vi "Verarbeitung_Oben.vi"(8 "Fehler in":errorcluster, 10 "Größe Kontaktsuchfeld":sgl=50.0, 11 "Cluster in":T1={"Initialisierung"={"Online?"=FALSE, "Grundpfad"=path "", "Kamera Oben"="", "IP-Adresse Flüssiglinse"="", "Flüssiglinse"=refnum, "Kamera Unten"="", "IP-Adresse SPS"="", "SPS-Verbindung"={"TCP Connection Ref"=refnum, "IP address"="", "timeout ms"=5000, "Connected?"=FALSE, "PLC Type"=enum."S7 1200", "Rack S7 400"=0, "Slot S7 400"=0, "PDU Size"=0, "connection semaphore"=refnum}, "IP-Adresse Lichtgitter"="", "Lichtgitter"=refnum, "Skalierungsfaktor"=0.0, "Bilder Oben"=[], "Bild Unten"=refnum, "Bild Ausschnitt Unten"=refnum}, "Einstellungen"={"Gesamtablauf gestartet"=FALSE, "i. O. Bilder speichern"=FALSE, "Bildspeicherung Offline"=FALSE, "Ausgewähltes Offline-Datum"="", "Ausgewähltes Offline-Teil"="", "Speicherpfad Bilder"=path ""}, "Artikeldaten"={"Artikelnummer"="", "Fertigungsauftrag"="", "Muster ISO"=refnum, "Belichtungszeit Referenzmarken"=0.0, "Fokus Referenzmarken"=0.0, "Belichtungszeit ISO"=0.0, "Fokus ISO"=0.0, "Belichtungszeit Unten"=0.0, "Kontaktanzahl"=0, "Aktueller Kontakt"=0, "Kontaktposition"={"x"=0.0, "y"=0.0}, "Winkel ISO"=0.0, "ISO-Muster nicht vorhanden"=FALSE}, "Werte Kamera Oben"={"Koordinatensystem"={"Punkt x-Achse"={"X"=0.0, "Y"=0.0}, "Ursprung"={"X"=0.0, "Y"=0.0}, "Punkt y-Achse"={"X"=0.0, "Y"=0.0}}, "Position Kontakt"={"x"=0.0, "y"=0.0}, "Winkel Kontakt"=0.0}, "Werte Kamera Unten"={"Prüfung Unten n. i. O."=FALSE}, "Werte Lichtgitter"={"Messwerte Referenzmarken"=[], "Mittelpunkt Referenzmarken"={"x"=0.0, "y"=0.0}, "Messwerte Kontakt"=[], "Offset"={"x"=0.0, "y"=0.0}}, "Rückmeldungen"={"Koordinaten ermittelt"=FALSE, "Vermessung Lichtgitter fertig"=FALSE, "Nachkontrolle Kamera Unten fertig"=FALSE}, "Fehler"={"Referenzen nicht gefunden"=FALSE, "Kontakt nicht gefunden"=FALSE, "Referenzen nicht in Lichtgitter"=FALSE, "Kontakt zu groß"=FALSE, "Kontakt zu klein"=FALSE}, "Statistik"={"Statistiken"=[]}, "Timer"={"Timer Start Position"=0, "Timer Start Lichtgitter"=0, "Timer Start Kamera Unten"=0}}) -> (0 "Fehler out":errorcluster, 2 "Durchmesser Loch":dbl, 3 "Cluster out":T1={"Initialisierung"={"Online?"=FALSE, "Grundpfad"=path "", "Kamera Oben"="", "IP-Adresse Flüssiglinse"="", "Flüssiglinse"=refnum, "Kamera Unten"="", "IP-Adresse SPS"="", "SPS-Verbindung"={"TCP Connection Ref"=refnum, "IP address"="", "timeout ms"=5000, "Connected?"=FALSE, "PLC Type"=enum."S7 1200", "Rack S7 400"=0, "Slot S7 400"=0, "PDU Size"=0, "connection semaphore"=refnum}, "IP-Adresse Lichtgitter"="", "Lichtgitter"=refnum, "Skalierungsfaktor"=0.0, "Bilder Oben"=[], "Bild Unten"=refnum, "Bild Ausschnitt Unten"=refnum}, "Einstellungen"={"Gesamtablauf gestartet"=FALSE, "i. O. Bilder speichern"=FALSE, "Bildspeicherung Offline"=FALSE, "Ausgewähltes Offline-Datum"="", "Ausgewähltes Offline-Teil"="", "Speicherpfad Bilder"=path ""}, "Artikeldaten"={"Artikelnummer"="", "Fertigungsauftrag"="", "Muster ISO"=refnum, "Belichtungszeit Referenzmarken"=0.0, "Fokus Referenzmarken"=0.0, "Belichtungszeit ISO"=0.0, "Fokus ISO"=0.0, "Belichtungszeit Unten"=0.0, "Kontaktanzahl"=0, "Aktueller Kontakt"=0, "Kontaktposition"={"x"=0.0, "y"=0.0}, "Winkel ISO"=0.0, "ISO-Muster nicht vorhanden"=FALSE}, "Werte Kamera Oben"={"Koordinatensystem"={"Punkt x-Achse"={"X"=0.0, "Y"=0.0}, "Ursprung"={"X"=0.0, "Y"=0.0}, "Punkt y-Achse"={"X"=0.0, "Y"=0.0}}, "Position Kontakt"={"x"=0.0, "y"=0.0}, "Winkel Kontakt"=0.0}, "Werte Kamera Unten"={"Prüfung Unten n. i. O."=FALSE}, "Werte Lichtgitter"={"Messwerte Referenzmarken"=[], "Mittelpunkt Referenzmarken"={"x"=0.0, "y"=0.0}, "Messwerte Kontakt"=[], "Offset"={"x"=0.0, "y"=0.0}}, "Rückmeldungen"={"Koordinaten ermittelt"=FALSE, "Vermessung Lichtgitter fertig"=FALSE, "Nachkontrolle Kamera Unten fertig"=FALSE}, "Fehler"={"Referenzen nicht gefunden"=FALSE, "Kontakt nicht gefunden"=FALSE, "Referenzen nicht in Lichtgitter"=FALSE, "Kontakt zu groß"=FALSE, "Kontakt zu klein"=FALSE}, "Statistik"={"Statistiken"=[]}, "Timer"={"Timer Start Position"=0, "Timer Start Lichtgitter"=0, "Timer Start Kamera Unten"=0}})   [LabVIEW 2024]
doc: "Ermittelt die Position des nächsten Kontakts im Koordinatensystem der Referenzbohrungen."
uses:
  Cluster.ctl
  Kontaktmontagemodul.exe/1abvi3w/vi.lib/userDefined/High Color/IMAQdx.ctl
  Kontaktmontagemodul.exe/1abvi3w/vi.lib/DATA AHEAD/SP7/typedefs/S7 Connection.ctl
  Kontaktmontagemodul.exe/1abvi3w/vi.lib/DATA AHEAD/SP7/typedefs/PLC Type.ctl
  Kontaktmontagemodul.exe/1abvi3w/vi.lib/vision/Image Controls.llb/IMAQ Image.ctl
  Koordinatensystem.ctl
  Statistik.ctl
  Kontaktmontagemodul.exe/1abvi3w/vi.lib/DATA AHEAD/SP7/SP7.lvlib
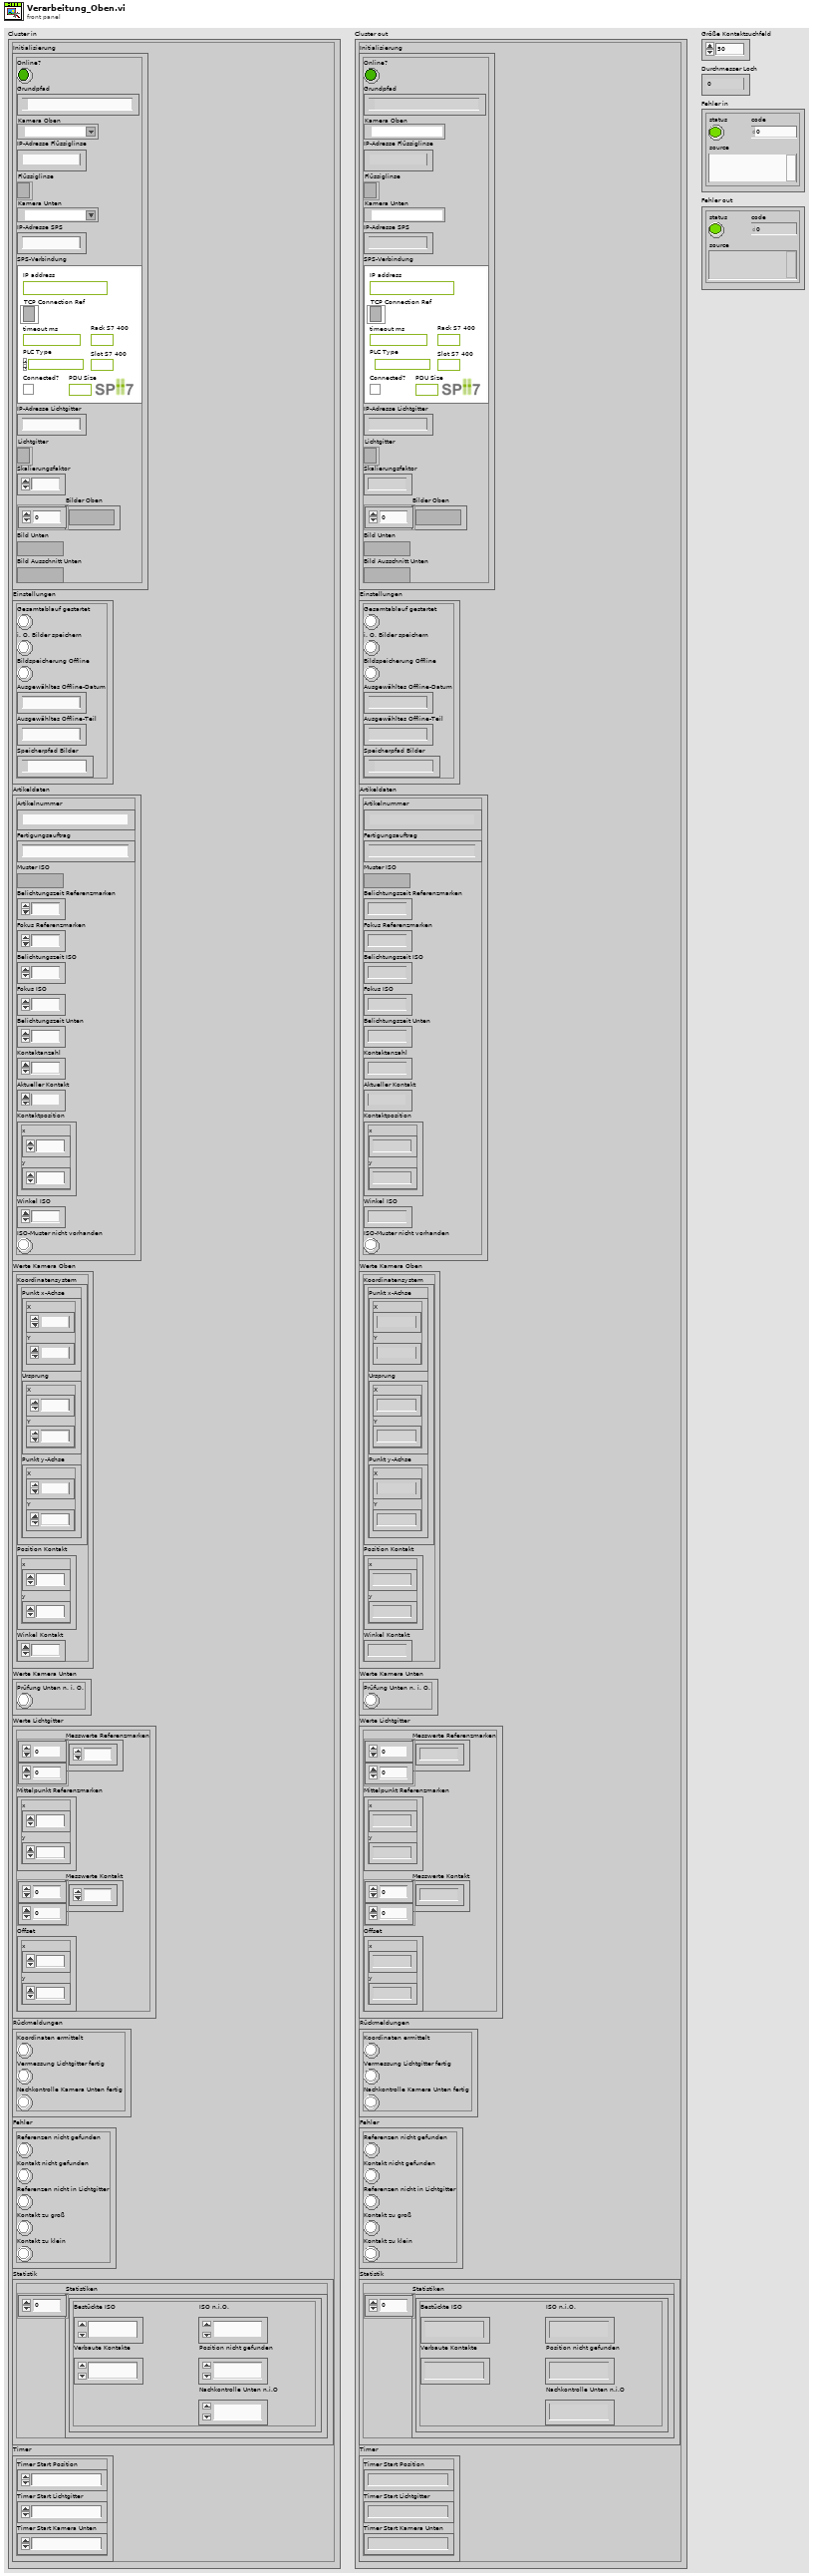
[diagram p1: front panel]
types:
  T1 = typedef "Cluster.ctl" = cluster{"Initialisierung":cluster{"Online?":bool, "Grundpfad":path, "Kamera Oben":T2, "IP-Adresse Flüssiglinse":string, "Flüssiglinse":refnum<k5>, "Kamera Unten":T2, "IP-Adresse SPS":string, "SPS-Verbindung":T3, "IP-Adresse Lichtgitter":string, "Lichtgitter":refnum<k5>, "Skalierungsfaktor":dbl, "Bilder Oben":T6[], "Bild Unten":T6, "Bild Ausschnitt Unten":T6}, "Einstellungen":cluster{"Gesamtablauf gestartet":bool, "i. O. Bilder speichern":bool, "Bildspeicherung Offline":bool, "Ausgewähltes Offline-Datum":string, "Ausgewähltes Offline-Teil":string, "Speicherpfad Bilder":path}, "Artikeldaten":cluster{"Artikelnummer":string, "Fertigungsauftrag":string, "Muster ISO":T6, "Belichtungszeit Referenzmarken":dbl, "Fokus Referenzmarken":dbl, "Belichtungszeit ISO":dbl, "Fokus ISO":dbl, "Belichtungszeit Unten":dbl, "Kontaktanzahl":u32, "Aktueller Kontakt":i16, "Kontaktposition":cluster{"x":sgl, "y":sgl}, "Winkel ISO":sgl, "ISO-Muster nicht vorhanden":bool}, "Werte Kamera Oben":cluster{"Koordinatensystem":T7, "Position Kontakt":cluster{"x":dbl, "y":dbl}, "Winkel Kontakt":dbl}, "Werte Kamera Unten":cluster{"Prüfung Unten n. i. O.":bool}, "Werte Lichtgitter":cluster{"Messwerte Referenzmarken":dbl[][], "Mittelpunkt Referenzmarken":cluster{"x":dbl, "y":dbl}, "Messwerte Kontakt":dbl[][], "Offset":cluster{"x":dbl, "y":dbl}}, "Rückmeldungen":cluster{"Koordinaten ermittelt":bool, "Vermessung Lichtgitter fertig":bool, "Nachkontrolle Kamera Unten fertig":bool}, "Fehler":cluster{"Referenzen nicht gefunden":bool, "Kontakt nicht gefunden":bool, "Referenzen nicht in Lichtgitter":bool, "Kontakt zu groß":bool, "Kontakt zu klein":bool}, "Statistik":cluster{"Statistiken":T8[]}, "Timer":cluster{"Timer Start Position":u32, "Timer Start Lichtgitter":u32, "Timer Start Kamera Unten":u32}}
  T2 = typedef "IMAQdx.ctl" = refnum<k21>
  T3 = typedef "SP7.lvlib/S7 Connection.ctl" = cluster{"TCP Connection Ref":refnum<k5>, "IP address":string, "timeout ms":i32, "Connected?":bool, "PLC Type":T4, "Rack S7 400":u8, "Slot S7 400":u8, "PDU Size":u16, "connection semaphore":T5}
  T4 = typedef "SP7.lvlib/PLC Type.ctl" = enum16{"S7 200", "S7 300/400", "S7 1200", "S7 1500", "LOGO!8"}
  T5 = typedef "Semaphore RefNum" = refnum<k1>
  T6 = typedef "IMAQ Image.ctl" = refnum<image>
  T7 = typedef "Koordinatensystem.ctl" = cluster{"Punkt x-Achse":cluster{"X":sgl, "Y":sgl}, "Ursprung":cluster{"X":sgl, "Y":sgl}, "Punkt y-Achse":cluster{"X":sgl, "Y":sgl}}
  T8 = typedef "Statistik.ctl" = cluster{"Bestückte ISO":u32, "Verbaute Kontakte":u32, "ISO n.i.O.":u32, "Nachkontrolle Unten n.i.O":u32, "Position nicht gefunden":u32}
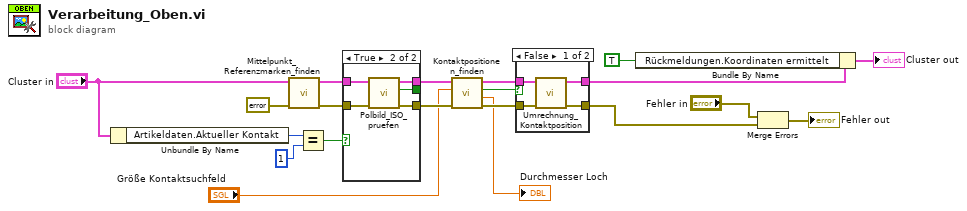
[diagram p0: block diagram]
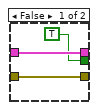
[diagram p2: hidden frame]
diagram:
  n1 = Unbundle By Name("Cluster in") -> ("Artikeldaten.Aktueller Kontakt"=w15:i16)
  n2 = call "Mittelpunkt_Referenzmarken_finden.vi"("Fehler in"=errorcluster {"status"=FALSE, "code"=0, "source"=""} ("error in (no error)"), "Cluster in"="Cluster in") -> ("Fehler out"=w9:errorcluster, "Cluster out"=w8:T1)  [unwired: 7 in, 1 out]
  n3 = Equal?(x=w15, y=i16 1) -> (x = y?=w3:bool)
  n4 = case shown="True" w3 {
    tunnel: w9 -> [w22 w28]
    tunnel: [w22 w27] -> w6
    tunnel: [w23 w26] -> w7
    tunnel: w8 -> [w23 w25]
    tunnel: [TRUE ("Poolbild ISO i.O.?") w24] -> _
    frame False {
    }
    frame True {
      n5 = call "Polbild_ISO_pruefen.vi"("Fehler in"=w28, "Cluster in"=w25) -> ("Fehler out"=w27:errorcluster, "Polbild i.O."=w24:bool, "Cluster out"=w26:T1)  [unwired: 7 in]
    }
  }
  n6 = call "Kontaktpositionen_finden.vi"("Fehler in"=w6, "Größe Kontaktsuchfeld"="Größe Kontaktsuchfeld", "Cluster in"=w7) -> ("Fehler out"=w11:errorcluster, "Durchmesser Loch"=→"Durchmesser Loch":dbl, "Kontakt nicht gefunden"=w10:bool, "Cluster out"=w12:T1)  [unwired: 5 in]
  n7 = case shown="False" w10 {
    tunnel: [w32 w33] -> w17
    tunnel: w12 -> [w31 w34]
    tunnel: w11 -> [w30 w33]
    tunnel: [w29 w34] -> w16
    frame False {
      n8 = call "Umrechnung_Kontaktposition.vi"("Fehler in"=w30, "Cluster in"=w31) -> ("Fehler out"=w32:errorcluster, "Cluster out"=w29:T1)  [unwired: 8 in]
    }
    frame True {
    }
  }
  n9 = Bundle By Name(cluster=w16, "Rückmeldungen.Koordinaten ermittelt"=TRUE ("Kamera Oben.Koordinaten ermittelt")) -> (→"Cluster out":T1)
  n10 = Merge Errors("Fehler in", w17) -> (→"Fehler out":errorcluster)
